vi "test type string.vi"() -> ()   [LabVIEW 2018, in "LV-Julia_ZMQ-Roundtrip_lib.lvlib"]
uses:
  LV-Julia_ZMQ-Roundtrip_lib.lvlib
panel:
  out "error out":errorcluster
  out "type string (7.x only)":i16[](array[numeric])
  out "converted":u8[](array[numeric])
  in  "Numeric":i32
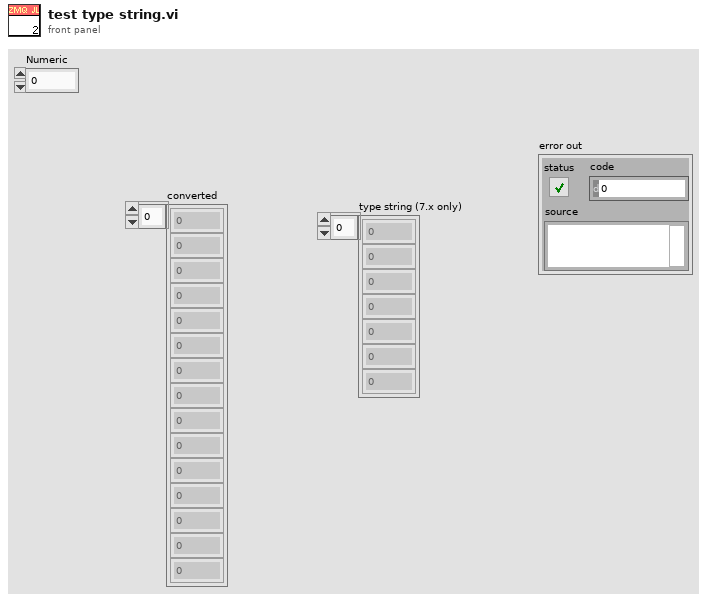
[diagram p1: front panel]
types:
  T1 = enum16{"big-endian, network order", "native, host order", "little-endian"}
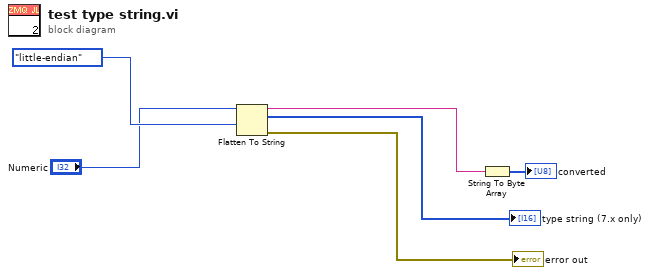
[diagram p0: block diagram]
diagram:
  n1 = Flatten To String(anything="Numeric", byte order (0:big-endian, network order)=T1."little-endian") -> (data string=w6:string, type string=→"type string (7.x only)":i16[], error out=→"error out":errorcluster)  [unwired: 2 in]
  n2 = String To Byte Array(string=w6) -> (unsigned byte array=→"converted":u8[])
